vi "GetMeasureLowRange.vi"(7 "SMU":T2, 8 "Error In":errorcluster, 10 "Range Function":T1, 11 "Kiethley 2602 In":refnum<visa-resource-name>) -> (0 "Error Out":errorcluster, 2 "Range (V or A)":dbl, 3 "Keithley 2602 Out":refnum<visa-resource-name>)   [LabVIEW 2012, in "Keithley-2602.lvlib"]
uses:
  Keithley-2602.lvlib
  Controls/SMU.ctl
  Controls/RangeFunction.ctl
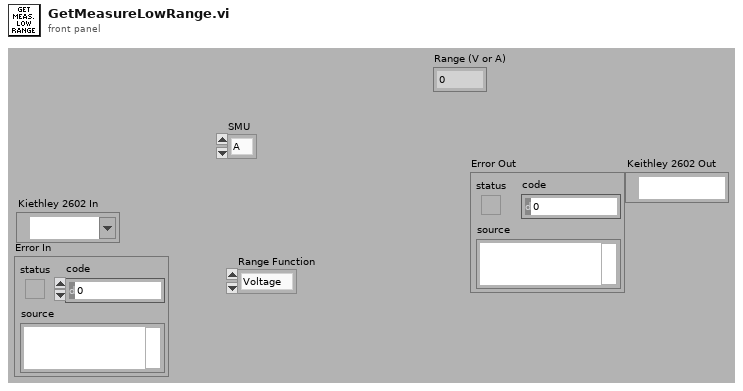
[diagram p1: front panel]
types:
  T1 = typedef "Keithley-2602.lvlib/RangeFunction.ctl" = enum16{"Voltage", "Current"}
  T2 = typedef "Keithley-2602.lvlib/SMU.ctl" = enum16{"A", "B"}
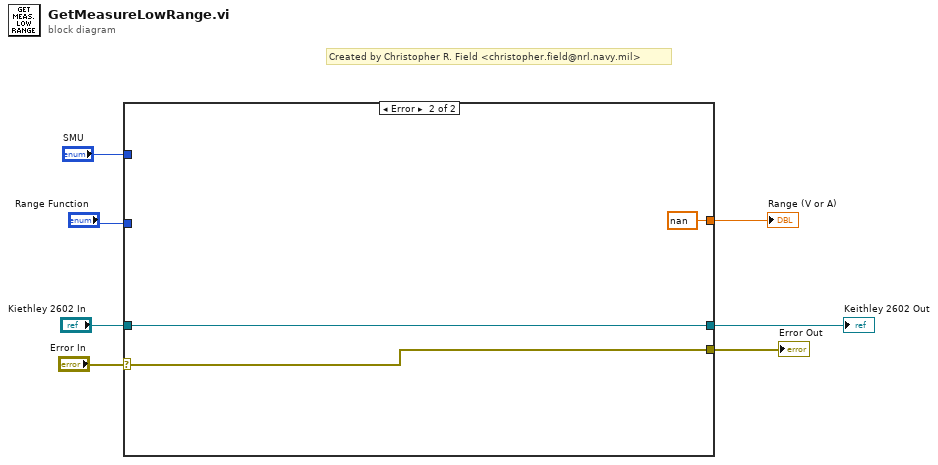
[diagram p0: block diagram]
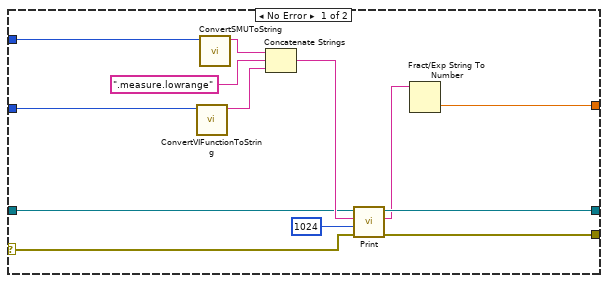
[diagram p2: hidden frame]
diagram:
  # "Created by Christopher R. Field <christopher.field@nrl.navy.mil>"
  n1 = case shown="Error" "Error In" {
    selector: "Error In" -> [w8 w22]
    tunnel: "Kiethley 2602 In" -> [w16 w23]
    tunnel: [w15 w22] -> w6
    tunnel: [w14 w23] -> w5
    tunnel: [w11 nan] -> w4
    tunnel: "SMU" -> [w10 _]
    tunnel: "Range Function" -> [w9 _]
    frame No Error {
      n2 = call "ConvertVIFunctionToString.vi"("Function"=w9) -> ("Function (v or i)"=w13:string)  [unwired: 10 in]
      n3 = call "ConvertSMUToString.vi"("SMU"=w10) -> ("Channel"=w20:string)  [unwired: 10 in]
      n4 = Concatenate Strings(w20, ".measure.lowrange", w13) -> (w18:string)
      n5 = call "Print.vi"("Error In"=w8, "Byte Count"=u32 1024, "Attribute"=w18, "Kiethley 2602 In"=w16) -> ("Error Out"=w15:errorcluster, "Output"=w12:string, "Keithley 2602 Out"=w14:refnum<visa-resource-name>)  [unwired: 5 in]
      n6 = Fract/Exp String To Number(string=w12) -> (number=w11:dbl)  [unwired: 3 in, 1 out]
    }
    frame Error {
    }
  }
  "Error Out" <- w6
  "Keithley 2602 Out" <- w5
  "Range (V or A)" <- w4
